vi "Construct Sequence.vi"(8 "error in":errorcluster, 11 "Schedule Builder in":refnum<class "Schedule Builder.lvclass">) -> (0 "error out":errorcluster, 2 "New Sequence":refnum<class "SEQ.lvclass">, 3 "Schedule Builder out":refnum<class "Schedule Builder.lvclass">)   [LabVIEW 2012, in "Schedule Builder.lvclass"]
doc: "Construct a new sequence using the builder class."
uses:
  Schedule Builder.lvclass
  MSR/Sequence Composition/SEQ/SEQ.lvclass
  Configuration Data/Task Data.lvclass
  Tasks.lvclass
  Type Defs/Mode Select.ctl
  Scheduler SEQ/Scheduler.lvclass
  MSR/Sequence Composition/Sequence Factory/Sequence Builder.lvclass/Sequence Builder.ctl
  Configuration Data/Task Data.lvclass/Task Data.ctl
  Schedule Builder.lvclass/Schedule Builder.ctl
  Tasks.lvclass/Tasks.ctl
  Scheduler SEQ/Scheduler.lvclass/Scheduler.ctl
  Configuration Data/Read Act Time.vi
  Configuration Data/Read Active.vi
  Configuration Data/Read Mode Select.vi
  Configuration Data/Read Altitude.vi
  MSR/Sequence Composition/Sequence Factory/Accessors/Read Config Data.vi
  Write UI Event.vi
  Scheduler SEQ/Write DOW.vi
  MSR/Base Data Class/Data.lvclass
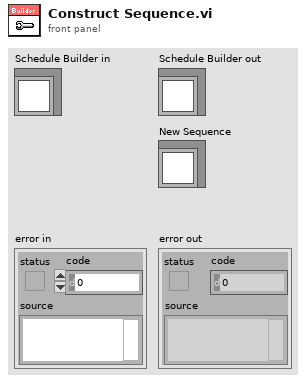
[diagram p1: front panel]
types:
  T1 = typedef "Mode Select.ctl" = enum8{"Off", "Stby", "Hold", "Run"}
  T2 = cluster{"Data Access:Active":bool, "Data Access:Act Time":sgl, "Data Access:Mode Select":T1, "Data Access:Altitude":dbl}
  T3 = typedef "LVDateTimeRec.ctl" = cluster{"fractional second":dbl, "second":i32, "minute":i32, "hour":i32, "day of month":i32, "month":i32, "year":i32, "day of week":i32, "day of year":i32, "DST":i32}
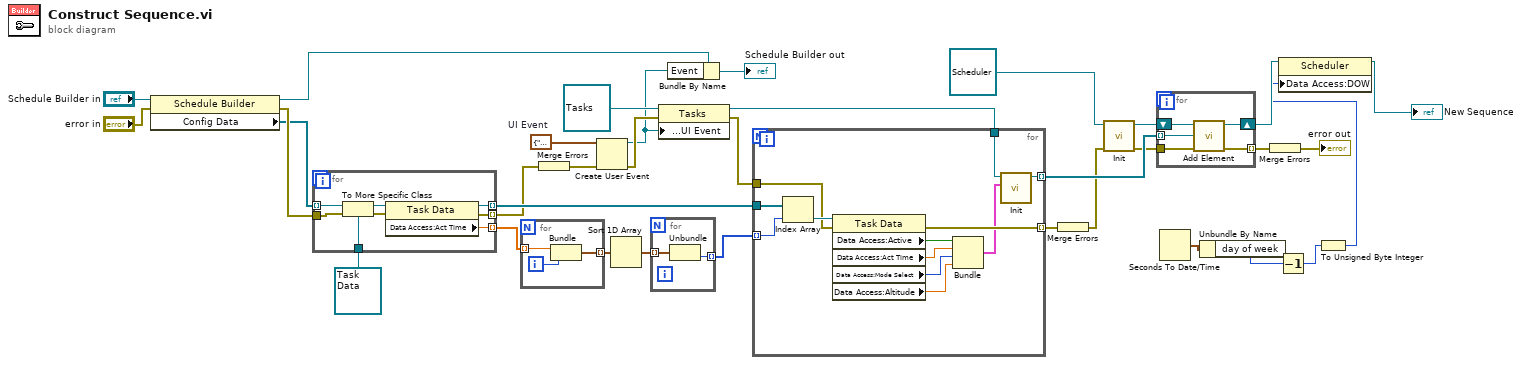
[diagram p0: block diagram]
diagram:
  w16 = cluster{"Mode Select":T1, "Altitude":sgl} {"Mode Select"=enum."Off", "Altitude"=0.0}  # UI Event
  n1 = property class="Schedule Builder"(reference="Schedule Builder in", error in="error in") -> (reference out=w13:refnum<class "Schedule Builder.lvclass">, error out=w31:errorcluster, "Config Data"=w30:refnum<class "Data.lvclass">[])
  n2 = for {
    tunnel: w30 -> [w42] mode=indexing
    tunnel: refnum<class "Task Data.lvclass"> refnum ("Task Data") -> [w41]
    tunnel: w31 -> [w40]
    tunnel: [w37] -> w2 mode=indexing
    tunnel: [w36] -> w29 mode=indexing
    tunnel: [w35] -> w28 mode=indexing
    n3 = To More Specific Class(target class=w41, reference=w42, error in=w40) -> (specific class reference=w39:refnum<class "Task Data.lvclass">, error out=w38:errorcluster)
    n4 = property class="Task Data"(reference=w39, error in=w38) -> (reference out=w36:refnum<class "Task Data.lvclass">, error out=w35:errorcluster, "Data Access:Act Time"=w37:sgl)
  }
  n5 = for {
    tunnel: w2 -> [w45] mode=indexing
    tunnel: [w43] -> w4 mode=indexing
    i -> [w44]
    n6 = Bundle("Data Access:Act Time"=w45, w44) -> (w43:cluster{"Data Access:Act Time":sgl, i32})  [unwired: 1 in]
  }
  n7 = Merge Errors(w28) -> (w25:errorcluster)
  n8 = Create User Event(user event datatype=w16, error in=w25) -> (user event=w11:refnum<user-event>, error out=w15:errorcluster)
  n9 = Sort 1D Array(array=w4) -> (sorted array=w3:cluster{"Data Access:Act Time":sgl, i32}[])
  n10 = for {
    tunnel: w3 -> [w47] mode=indexing
    tunnel: [w46] -> w1 mode=indexing
    n11 = Unbundle(w47) -> (w46:i32)  [unwired: 1 out]
  }
  n12 = property class="Tasks"(reference=refnum<class "Tasks.lvclass"> refnum ("Tasks"), error in=w15, "Data Access:UI Event"=w11) -> (reference out=w26:refnum<class "Tasks.lvclass">, error out=w14:errorcluster)
  n13 = Bundle By Name(cluster=w13, "Event"=w11) -> (→"Schedule Builder out":refnum<class "Schedule Builder.lvclass">)
  n14 = for {
    tunnel: w29 -> [w59]
    tunnel: w1 -> [w58] mode=indexing
    tunnel: w26 -> [w52]
    tunnel: w14 -> [w51]
    tunnel: [w50] -> w24 mode=indexing
    tunnel: [w49] -> w23 mode=indexing
    n15 = Index Array(array=w59, index=w58) -> (element=w57:refnum<class "Task Data.lvclass">)
    n16 = property class="Task Data"(reference=w57, error in=w51) -> (error out=w50:errorcluster, "Data Access:Active"=w56:bool, "Data Access:Act Time"=w55:sgl, "Data Access:Mode Select"=w54:T1, "Data Access:Altitude"=w53:dbl)  [unwired: 1 out]
    n17 = Bundle("Data Access:Active"=w56, "Data Access:Act Time"=w55, "Data Access:Mode Select"=w54, "Data Access:Altitude"=w53) -> (w48:T2)  [unwired: 1 in]
    n18 = call "Init.vi"("Init Data"=w48, "Tasks in"=w52) -> ("Tasks out"=w49:refnum<class "Tasks.lvclass">)  [unwired: 9 in]
  }
  n19 = Merge Errors(w24) -> (w18:errorcluster)
  n20 = call-dynamic "Init.vi"("error in"=w18, "SEQ in"=refnum<class "Scheduler.lvclass"> refnum ("Scheduler")) -> ("error out"=w17:errorcluster, "SEQ out"=w22:refnum<class "Scheduler.lvclass">)  [unwired: 8 in]
  n21 = for {
    tunnel: w23 -> [w64] mode=indexing
    shift-right: [w62] -> w10
    shift-left: w22 -> [w63]
    tunnel: [w61] -> w20 mode=indexing
    tunnel: w17 -> [w60]
    n22 = call "Add Element.vi"("error in"=w60, "STEP"=w64, "SEQ in"=w63) -> ("error out"=w61:errorcluster, "SEQ out"=w62:refnum<class "Scheduler.lvclass">)  [unwired: 7 in]
  }
  n23 = Seconds To Date/Time() -> (date time rec=w8:T3)  [unwired: 2 in]
  n24 = Unbundle By Name(w8) -> ("day of week"=w5:i32)
  n25 = Merge Errors(w20) -> (→"error out":errorcluster)
  n26 = Decrement(x=w5) -> (x-1=w6:i32)
  n27 = To Unsigned Byte Integer(number=w6) -> (unsigned 8bit integer=w7:u8)
  n28 = property class="Scheduler"(reference=w10, "Data Access:DOW"=w7) -> (reference out=→"New Sequence":refnum<class "Scheduler.lvclass">)  [unwired: 1 in, 1 out]
